vi "load_setTorque.vi"(8 "error in (no error)":errorcluster, 10 "torque set":dbl, 11 "Instrument in":refnum<class "Instrument.lvclass">) -> (0 "error out":errorcluster, 3 "Instrument out":refnum<class "Instrument.lvclass">)   [LabVIEW 2019, in "Instrument.lvclass"]
uses:
  Instrument.lvclass
  Instrument.lvclass/Instrument.ctl
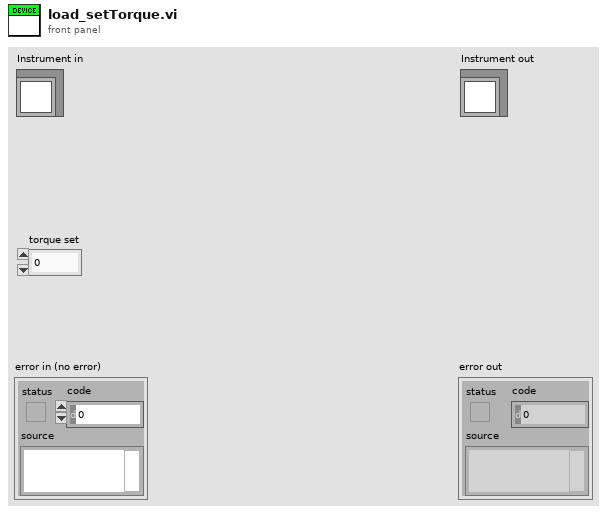
[diagram p1: front panel]
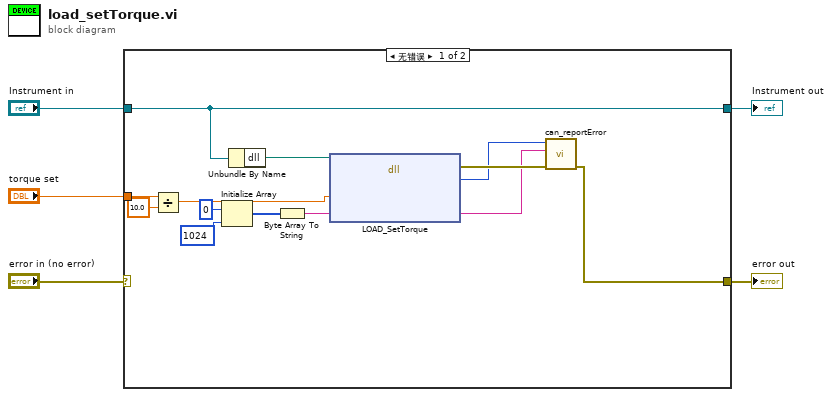
[diagram p0: block diagram]
diagram:
  n1 = case shown="无错误" "error in (no error)" {
    selector: "error in (no error)" -> [_ w20]
    tunnel: [w13 w20] -> w4
    tunnel: [w18 w19] -> w2
    tunnel: "Instrument in" -> [w18 w19]
    tunnel: "torque set" -> [w8 _]
    frame No Error {
      n2 = Divide(x=w8, y=10.0) -> (x/y=w6:dbl)
      n3 = Initialize Array(u8 0 ("element"), 1024 ("dimension size")) -> (w10:u8[])
      n4 = Unbundle By Name(w18) -> ("dll"=w17:path)
      n5 = Byte Array To String(unsigned byte array=w10) -> (string=w9:string)
      n6 = dll-call lib="C:/Dev/22KW-Dyno/software/data/DynoAPI.dll" fn="LOAD_SetTorque"(path in=w17, "torque"=w6, "errorMsg"=w9) -> (error out=w16:errorcluster, "return type"=w15:i32, "errorMsg"=w14:string)  [unwired: 3 in, 1 out]
      n7 = call "can_reportError.vi"("error in (no error)"=w16, "errorMsg"=w14, "return type"=w15) -> ("error out"=w13:errorcluster)  [unwired: 8 in]
    }
    frame Error {
    }
  }
  "error out" <- w4
  "Instrument out" <- w2
